vi "Write Build Directory.vi"(5 "Build Directory":path, 9 "PythonConverter_BD in":refnum<class "PyConvBD.lvclass">) -> (3 "PythonConverter_BD out":refnum<class "PyConvBD.lvclass">)   [LabVIEW 2014, in "Raspberry Pi Compatible Compiler for LabVIEW.lvlib" / "PyConvBD.lvclass"]
uses:
  PyConvBD.lvclass
  PyConvBD.lvclass/PyConvBD.ctl
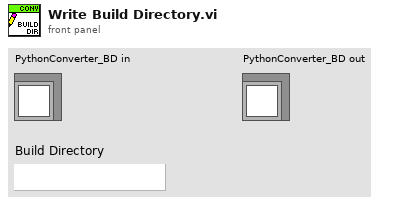
[diagram p1: front panel]
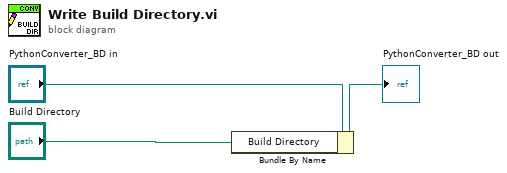
[diagram p0: block diagram]
diagram:
  n1 = Bundle By Name(cluster="PythonConverter_BD in", "Build Directory"="Build Directory") -> (→"PythonConverter_BD out":refnum<class "PyConvBD.lvclass">)
